vi "S2C_PCIe1762H_Proc_Initialize.vi"(8 "Error In":errorcluster, 11 "Initialize":string) -> (0 "Error Out":errorcluster)   [LabVIEW 2024]
uses:
  S2C_PCIe1762H_Proc_Globals.vi
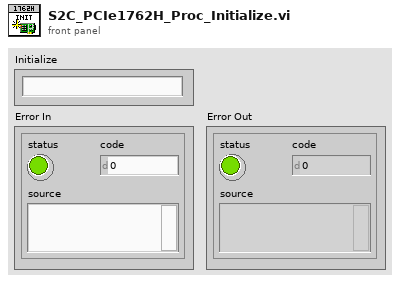
[diagram p1: front panel]
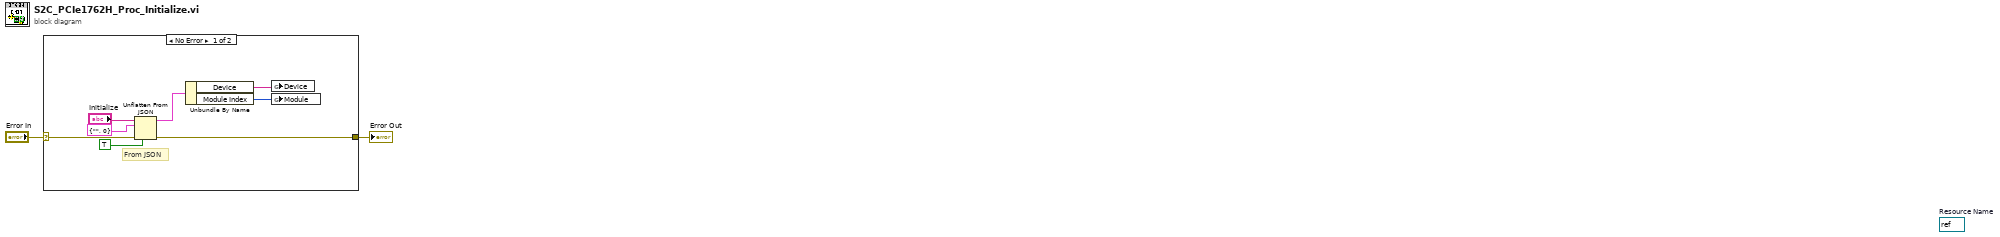
[diagram p0: block diagram]
diagram:
  (unwired) refnum<visa-resource-name> refnum  # Resource Name
  n1 = case shown="No Error" "Error In" {
    selector: "Error In" -> [w7 w11]
    tunnel: [w4 w11] -> w1
    frame No Error {
      # "From JSON"
      n2 = Unflatten From JSON(JSON string="Initialize", type and defaults=cluster{"Device":string, "Module Index":i32} {"Device"="", "Module Index"=0}, default null elements? (F)=TRUE, error in (no error)=w7) -> (value=w10:cluster{"Device":string, "Module Index":i32}, error out=w4:errorcluster)  [unwired: 3 in]
      n3 = Unbundle By Name(w10) -> ("Device"=w5:string, "Module Index"=w3:i32)
      n4 = global write "S2C_PCIe1762H_Proc_Globals.vi" "Device"(w5) -> ()
      n5 = global write "S2C_PCIe1762H_Proc_Globals.vi" "Module"(w3) -> ()
    }
    frame Error {
    }
  }
  "Error Out" <- w1
